vi "FlatToRichni_protobuf_types_WaveformAttributeValue.vi"(5 "OutputClusterType":T1, 11 "InputCluster":T2) -> (3 "OutputCluster":T1)   [LabVIEW 2021, in "ni.protobuf.types.lvlib"]
uses:
  ni.protobuf.types.lvlib
  ni_protobuf_types_WaveformAttributeValue_Flat.ctl
  ni_protobuf_types_WaveformAttributeValue.ctl
  ni_protobuf_types_WaveformAttributeValue_attribute/ni_protobuf_types_WaveformAttributeValue_attribute.lvclass
  ni_protobuf_types_WaveformAttributeValue_attribute/ni_protobuf_types_WaveformAttributeValue_attribute.lvclass/ni_protobuf_types_WaveformAttributeValue_attribute.ctl
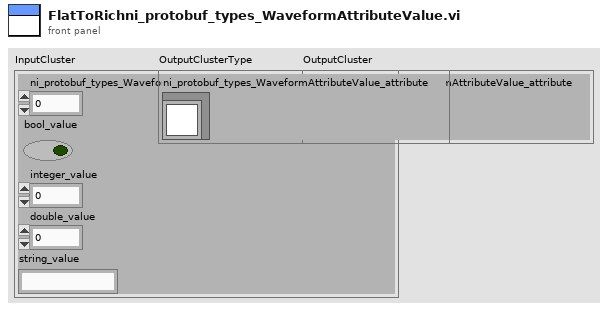
[diagram p1: front panel]
types:
  T1 = typedef "ni.protobuf.types.lvlib/ni_protobuf_types_WaveformAttributeValue.ctl" = cluster{"ni_protobuf_types_WaveformAttributeValue_attribute":refnum<class "ni_protobuf_types_WaveformAttributeValue_attribute.lvclass">}
  T2 = typedef "ni.protobuf.types.lvlib/ni_protobuf_types_WaveformAttributeValue_Flat.ctl" = cluster{"ni_protobuf_types_WaveformAttributeValue_attribute_selected_index":i32, "bool_value":bool, "integer_value":i32, "double_value":dbl, "string_value":string}
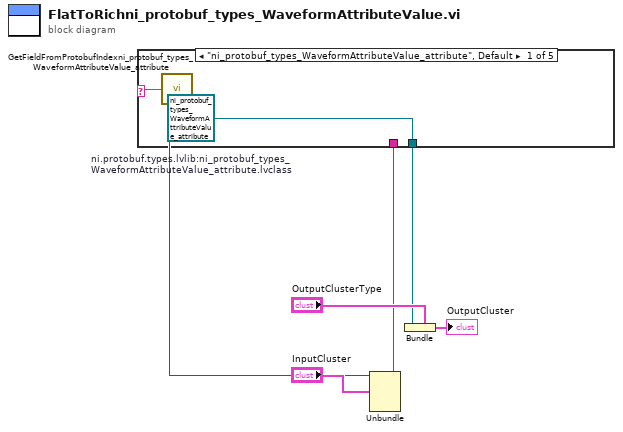
[diagram p0: block diagram]
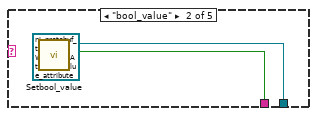
[diagram p2: hidden frame]
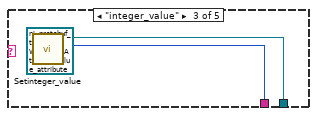
[diagram p3: hidden frame]
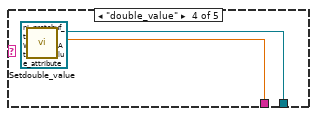
[diagram p4: hidden frame]
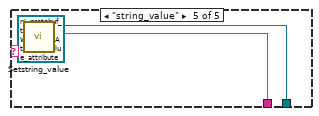
[diagram p5: hidden frame]
diagram:
  n1 = Unbundle "Unbundle"("InputCluster") -> ("ni_protobuf_types_WaveformAttributeValue_attribute_selected_index"=w7:i32, "bool_value"=w4:bool, "integer_value"=w3:i32, "double_value"=w2:dbl, "string_value"=w1:string)
  n2 = call "GetFieldFromProtobufIndexni_protobuf_types_WaveformAttributeValue_attribute.vi"("protobuf index"=w7) -> ("oneof field name"=w6:string)
  n3 = case "ni_protobuf_types_WaveformAttributeValue_attribute" shown="\"ni_protobuf_types_WaveformAttributeValue_attribute\", Default" w6 {
    tunnel: [w11 w13 w16 w19 w22] -> w5
    tunnel: w4 -> [_ w14 _ _ _]
    tunnel: w3 -> [_ _ w17 _ _]
    tunnel: w2 -> [_ _ _ w20 _]
    tunnel: w1 -> [_ _ _ _ w23]
    frame "ni_protobuf_types_WaveformAttributeValue_attribute", Default {
      w11 = refnum<class "ni_protobuf_types_WaveformAttributeValue_attribute.lvclass"> refnum  # ni.protobuf.types.lvlib:ni_protobuf_types_WaveformAttributeValue_attribute.lvclass
    }
    frame "bool_value" {
      n4 = call "Setbool_value.vi"("Set_Val"=w14, "OneOfTemplate in"=refnum<class "ni_protobuf_types_WaveformAttributeValue_attribute.lvclass"> refnum) -> ("OneOfTemplate out"=w13:refnum<class "ni_protobuf_types_WaveformAttributeValue_attribute.lvclass">)  [unwired: 8 in, 1 out]
    }
    frame "integer_value" {
      n5 = call "Setinteger_value.vi"("Set_Val"=w17, "OneOfTemplate in"=refnum<class "ni_protobuf_types_WaveformAttributeValue_attribute.lvclass"> refnum) -> ("OneOfTemplate out"=w16:refnum<class "ni_protobuf_types_WaveformAttributeValue_attribute.lvclass">)  [unwired: 8 in, 1 out]
    }
    frame "double_value" {
      n6 = call "Setdouble_value.vi"("Set_Val"=w20, "OneOfTemplate in"=refnum<class "ni_protobuf_types_WaveformAttributeValue_attribute.lvclass"> refnum) -> ("OneOfTemplate out"=w19:refnum<class "ni_protobuf_types_WaveformAttributeValue_attribute.lvclass">)  [unwired: 8 in, 1 out]
    }
    frame "string_value" {
      n7 = call "Setstring_value.vi"("Set_Val"=w23, "OneOfTemplate in"=refnum<class "ni_protobuf_types_WaveformAttributeValue_attribute.lvclass"> refnum) -> ("OneOfTemplate out"=w22:refnum<class "ni_protobuf_types_WaveformAttributeValue_attribute.lvclass">)  [unwired: 8 in, 1 out]
    }
  }
  n8 = Bundle "Bundle"(cluster="OutputClusterType", "ni_protobuf_types_WaveformAttributeValue_attribute"=w5) -> (→"OutputCluster":T1)
